vi "BRig_dataAnalog_valueAI0_1.vi"() -> (2 "output_valueAI0_1":i32)   [LabVIEW 2014]
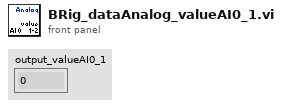
[diagram p1: front panel]
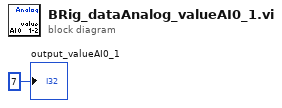
[diagram p0: block diagram]
diagram:
  "output_valueAI0_1" <- 7 ("output_iBlock")
